vi "XNET TCP Socket Wait on Listener.vi"(8 "error in":errorcluster, 9 "timeout ms (forever: -1)":i32=-1, 11 "listener socket in":refnum<k20>) -> (0 "error out":errorcluster, 1 "remote port":u16, 2 "remote address":string, 3 "listener socket out":refnum<k20>, 4 "connection socket":refnum<k20>)   [LabVIEW 2018]
doc: "Waits for an accepted TCP network connection."
uses:
  nixlvapi.dll
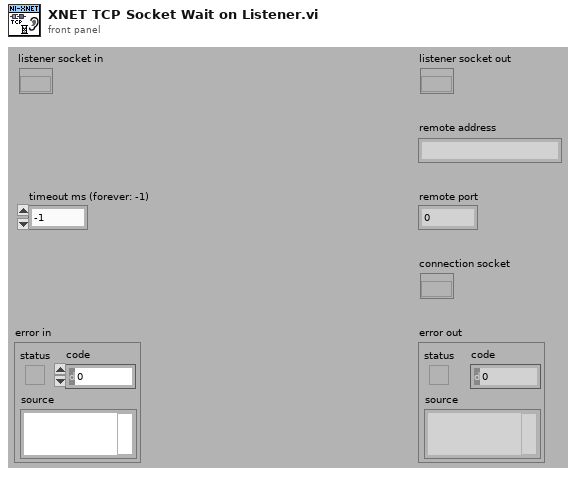
[diagram p1: front panel]
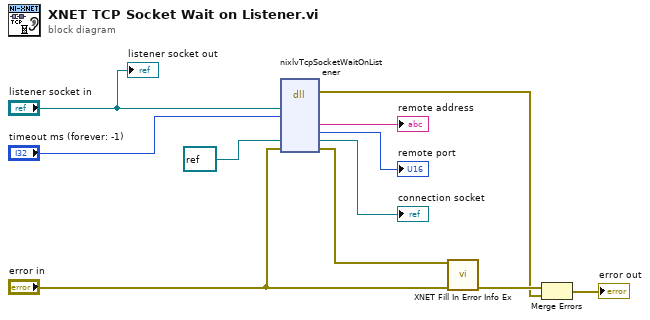
[diagram p0: block diagram]
diagram:
  n1 = dll-call lib="nixlvapi.*" fn="nixlvTcpSocketWaitOnListener" label="Call Library"("socketRef"="listener socket in", "timeoutMs"="timeout ms (forever: -1)", "connectionSocketRefObjPtr"=refnum<k20> refnum ("connection socket"), "errorInOut"="error in") -> (error out=w9:errorcluster, "remoteAddress"=→"remote address":string, "remotePort"=→"remote port":u16, "connectionSocketRefObjPtr"=→"connection socket":refnum<k20>, "errorInOut"=w11:errorcluster)  [unwired: 3 in, 6 out]
  n2 = call "XNET Fill In Error Info Ex.vi"("error xnet"=w11, "error in"="error in") -> ("error out"=w10:errorcluster)  [unwired: 13 in]
  n3 = Merge Errors(w10, w9) -> (→"error out":errorcluster)
  "listener socket out" <- "listener socket in"
